vi "_ExecuteInstruction.vi"(2 "Telemetry":refnum<k21>, 4 "Instructions":refnum<k21>, 5 "Output":refnum<k21>, 6 "error in (no error)":errorcluster, 7 "DebugOut":refnum<k21>, 8 "Port":T1="Mod6\\Port1", 9 "MPU in":refnum<class "MPU.lvclass">) -> (0 "error out":errorcluster, 1 "End Loop":bool, 3 "MPU out":refnum<class "MPU.lvclass">)   [LabVIEW 2018, in "Modbus_Processing_Unit.lvlib" / "MPU.lvclass"]
uses:
  MPU.lvclass
  PortType.ctl
  MPU.lvclass/MPU.ctl
  <vilib>/rvi/DataTransferAndStorage/Container/Common/niFpgaContainerExecOnDevCompGetState.vi
  <vilib>/rvi/Emulation/niFpgaEmulationIsFPGAContextNoSignature.vi
  <vilib>/rvi/DataTransferAndStorage/Container/Common/niFpgaContainerGetUniqueNameForEmu.vi
  <vilib>/rvi/Emulation/niFpgaProcessEmulError.vi
  <vilib>/rvi/Emulation/niFpgaSctlEmulationGetInTimedLoop.vi
  <vilib>/rvi/errors/nirviReportUnexpectedCaseInternalError (U32).vi
  <vilib>/rvi/Memory/Memory_Emulation/niFpgaMemoryEmulationCacheClearOnFirstRun.vi
  <vilib>/rvi/Memory/Memory_Emulation/nirvimemoryEmulationManagerCache_MakeExclusive.vi
  <vilib>/rvi/Memory/Memory_Emulation/niFpgaMemoryEmulationValidateCache.vi
  <vilib>/rvi/Memory/Memory_Emulation/nirvimemoryEmulationManagerCache_InsertValue.vi
  <vilib>/Utility/error.llb/Clear Errors.vi
  <vilib>/rvi/Memory/Memory_Emulation/nirvimemoryEmulationManagerCache_ReleaseExclusive.vi
  <vilib>/rvi/Memory/Memory_Emulation/nirvimemoryEmulationManagerCache_GetValue.vi
  <vilib>/rvi/Memory/Memory_Emulation/nirvimemoryEmulationManagerCache_SetValue.vi
  <vilib>/rvi/Emulation/niFpgaSctlEmulationResourceMgr.vi
  <vilib>/rvi/errors/niFpgaSetErrorForExecOnDevCompSimple.vi
  <vilib>/rvi/eio/common/nirviEmuReportErrorAndStop.vi
  <vilib>/rvi/FIFO/Fifo_Resource/nirvififoEmulationSetSize.vi
  <vilib>/rvi/FIFO/Fifo_Resource/nirviFifoEmulationQueueMgr.vi
  <instcachedir>/0/nirviFifoEmulationQueueMgr_E5CAEC123FF24DC58D834DCA3CDAA9B5.lvgen/nirviFifoEmulationQueueMgr_E5CAEC123FF24DC58D834DCA3CDAA9B5_001.vi
  <vilib>/rvi/FIFO/Fifo_Resource/nirvififoEmulationDetermineInputValidOut.vi
  <vilib>/rvi/FIFO/Fifo_Resource/nirvififoEmulationCreateLock.vi
  <vilib>/rvi/FIFO/Fifo_Resource/nirvififoEmulationObtainLock.vi
  <vilib>/rvi/FIFO/Fifo_Resource/nirvififoEmulationReleaseLock.vi
  <vilib>/rvi/occurrence/nirviWaitOnOccurrenceBase.vi
  <vilib>/rvi/errors/nirviReportUnexpectedCaseInternalError.vi
  <vilib>/rvi/interface/RandomDataEmulation/niFpgaRandomDataHandleErrors.vi
  <vilib>/rvi/DataTransferAndStorage/Container/XNode/niFpgaContainer.xnode
  <vilib>/rvi/Memory/Memory_Emulation/niFpgaMemoryEmulationRefIn.vi
  <vilib>/rvi/FIFO/Fifo_Resource/niFpgaFifoEmulationRefIn.vi
panel:
  # "Excutes a single instruction. Modify IP as needed. Signal if \ninstruction reading loop shall end in End Loop indicator."
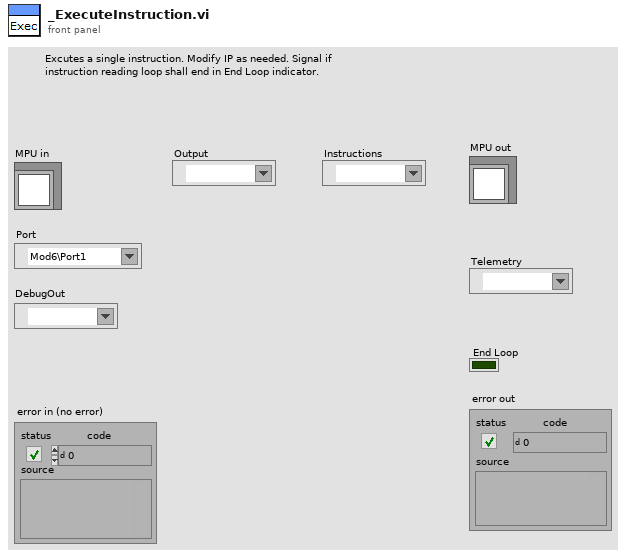
[diagram p1: front panel]
types:
  T1 = typedef "PortType.ctl" = refnum<k21>
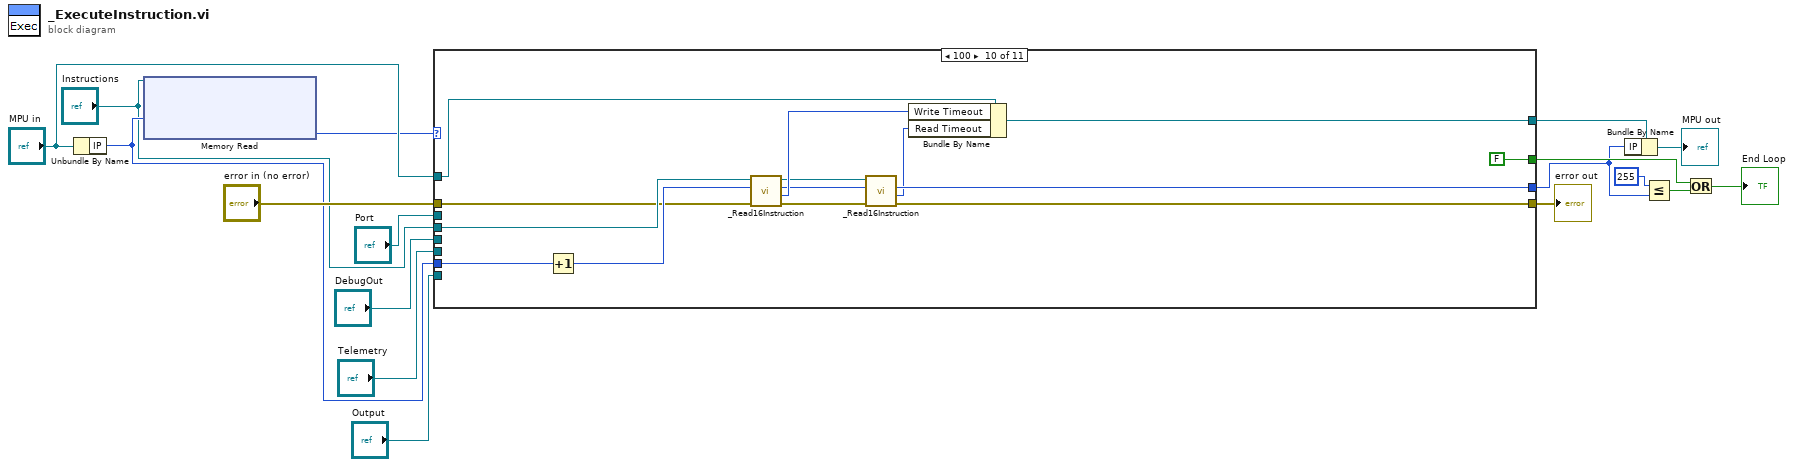
[diagram p0: block diagram]
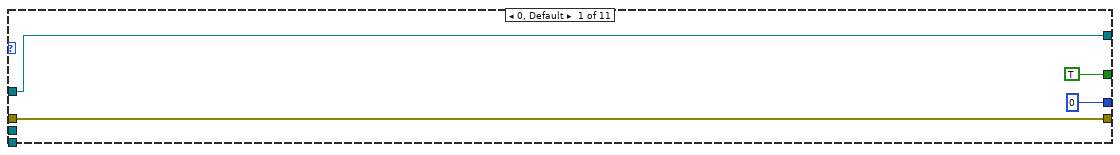
[diagram p2: hidden frame]
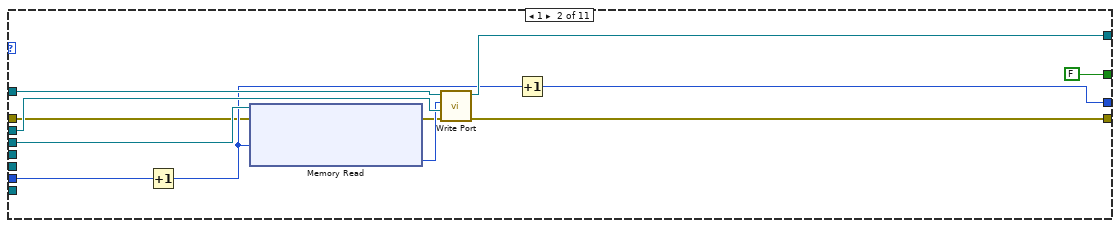
[diagram p3: hidden frame]
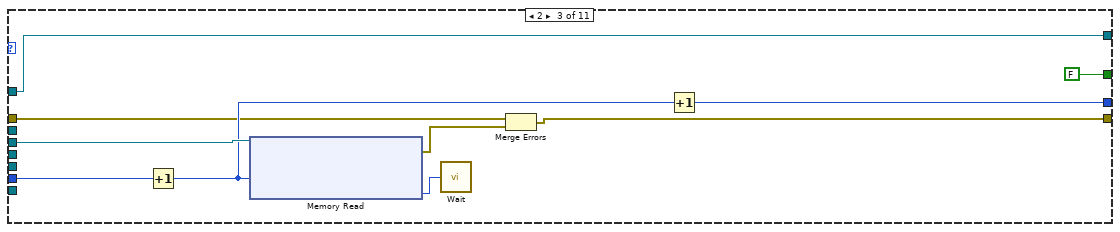
[diagram p4: hidden frame]
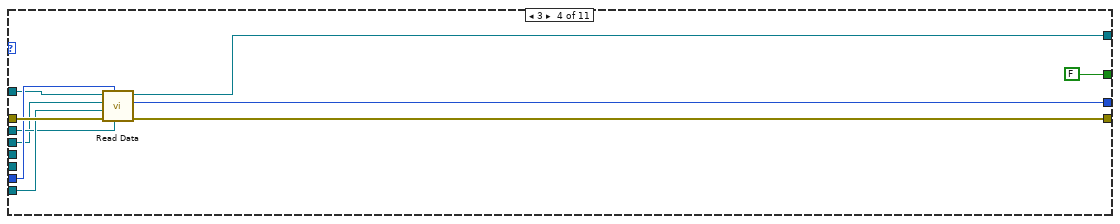
[diagram p5: hidden frame]
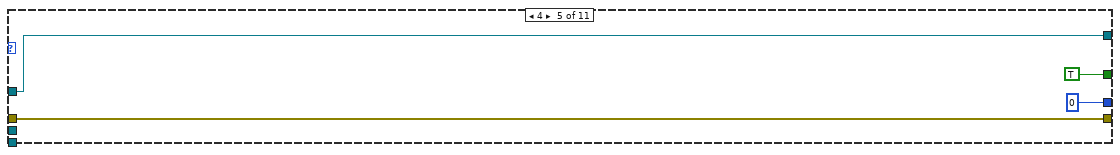
[diagram p6: hidden frame]
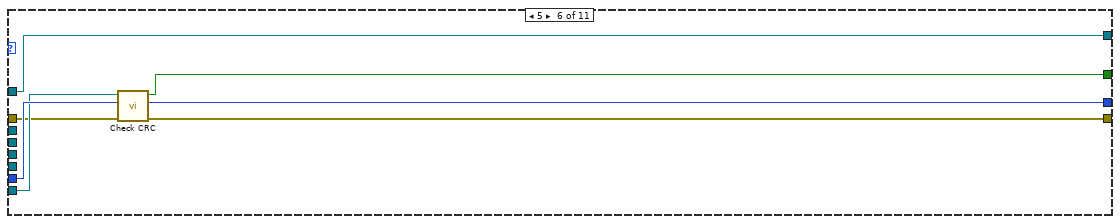
[diagram p7: hidden frame]
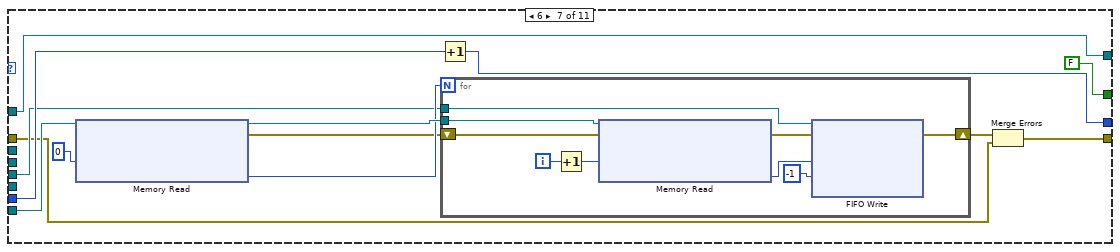
[diagram p8: hidden frame]
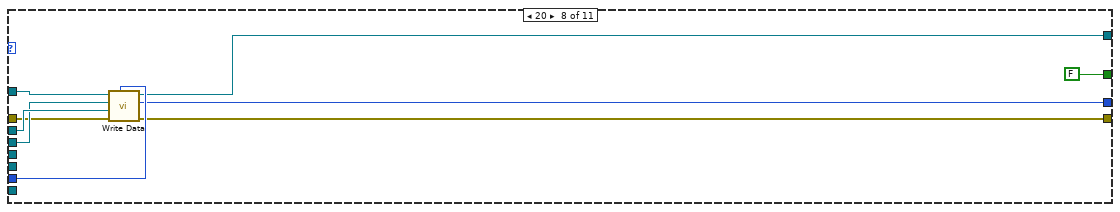
[diagram p9: hidden frame]
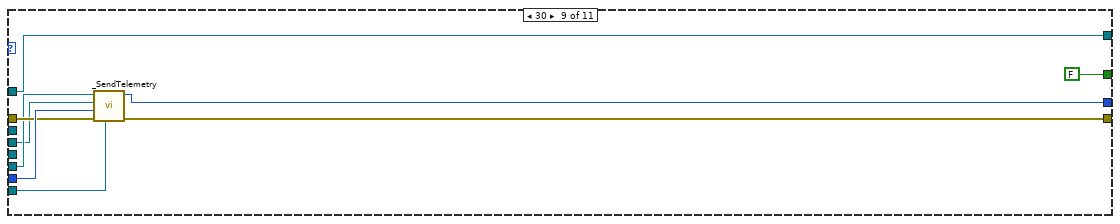
[diagram p10: hidden frame]
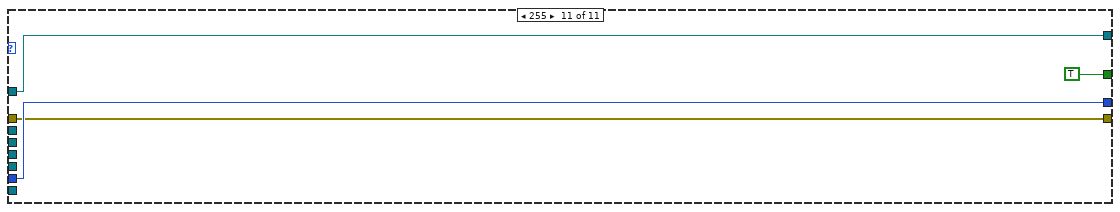
[diagram p11: hidden frame]
diagram:
  n1 = Unbundle By Name("MPU in") -> ("IP"=w5:i16)
  n2 = xnode ("Memory Read")("Address"=w5, "Memory In"="Instructions") -> ("Data"=w4:u8)  [unwired: 1 out]
  n3 = case shown="100" w4 {
    tunnel: [TRUE FALSE FALSE FALSE TRUE w60 FALSE FALSE FALSE FALSE ("Button") TRUE] -> w11
    tunnel: "error in (no error)" -> [w20 w23 w34 w52 w55 w58 w67 w89 w100 w112 w119]
    tunnel: w5 -> [_ w32 w43 w51 _ w63 w76 w94 w101 w116 w121]
    tunnel: [i16 0 ("IP") w31 w42 w53 i16 0 w62 w75 w92 w99 w108 w121] -> w10
    tunnel: "Output" -> [_ _ _ w49 _ w59 w73 _ w96 _ _]
    tunnel: [w20 w28 w35 w48 w55 w61 w68 w88 w103 w105 w119] -> w16
    tunnel: "MPU in" -> [w19 w30 w40 w46 w54 w64 w74 w95 w104 w118 w122]
    tunnel: [w19 w29 w40 w47 w54 w64 w74 w87 w104 w115 w122] -> w14
    tunnel: "Telemetry" -> [_ _ _ _ _ _ _ _ w98 _ _]
    tunnel: "Port" -> [_ w27 _ w45 _ _ _ w91 _ _ _]
    tunnel: "Instructions" -> [_ w26 w39 w44 _ _ _ w90 w97 w114 _]
    tunnel: "DebugOut" -> [_ _ _ _ _ _ w69 _ _ _ _]
    frame 0, Default {
    }
    frame 1 {
      n4 = Increment(x=w32) -> (x+1=w25:i16)
      n5 = xnode ("Memory Read")("Address"=w25, "error in (no error)"=w23, "Memory In"=w26) -> ("Data"=w24:u8, "error out"=w22:errorcluster)  [unwired: 1 out]
      n6 = call-dynamic "Write Port.vi"("error in (no error)"=w22, "Port"=w27, "Data"=w24, "MPU in"=w30) -> ("error out"=w28:errorcluster, "MPU out"=w29:refnum<class "MPU.lvclass">)  [unwired: 5 in, 1 out]
      n7 = Increment(x=w25) -> (x+1=w31:i16)
    }
    frame 2 {
      n8 = Increment(x=w43) -> (x+1=w36:i16)
      n9 = xnode ("Memory Read")("Address"=w36, "Memory In"=w39) -> ("Data"=w37:u8, "error out"=w38:errorcluster)  [unwired: 1 in, 1 out]
      n10 = call "Wait"("Count(mSec)"=w37) -> ()  [unwired: 1 out]
      n11 = Merge Errors(w34, w38) -> (w35:errorcluster)
      n12 = Increment(x=w36) -> (x+1=w42:i16)
    }
    frame 3 {
      n13 = call-dynamic "Read Data.vi"("Port"=w45, "IP"=w51, "error in (no error)"=w52, "Output"=w49, "Instructions"=w44, "MPU in"=w46) -> ("error out"=w48:errorcluster, "IP Out"=w53:i16, "MPU out"=w47:refnum<class "MPU.lvclass">)  [unwired: 3 in]
    }
    frame 4 {
    }
    frame 5 {
      n14 = call "Check CRC.vi"("error in (no error)"=w58, "IP"=w63, "Refnum in"=w59) -> ("error out"=w61:errorcluster, "Numeric"=w62:i16, "Button"=w60:bool)  [unwired: 6 in]
    }
    frame 6 {
      n15 = xnode ("Memory Read")("Address"=u32 0, "Memory In"=w73) -> ("Data"=w70:u8, "error out"=w66:errorcluster, "Memory Out"=w71:refnum<k21>)  [unwired: 1 in]
      n16 = Increment(x=w76) -> (x+1=w75:i16)
      n17 = for {
        N: w70 -> [_]
        tunnel: w69 -> [w86]
        tunnel: w71 -> [w84]
        shift-right: [w78] -> w65
        shift-left: w66 -> [w80]
        i -> [w83]
        n18 = Increment(x=w83) -> (x+1=w82:i32)
        n19 = xnode ("Memory Read")("Address"=w82, "error in (no error)"=w80, "Memory In"=w84) -> ("Data"=w81:u8, "error out"=w79:errorcluster)  [unwired: 1 out]
        n20 = xnode ("FIFO Write")("Element"=w81, "Timeout"=-1, "error in (no error)"=w79, "FIFO In"=w86) -> ("error out"=w78:errorcluster)  [unwired: 2 out]
      }
      n21 = Merge Errors(w65, w67) -> (w68:errorcluster)
    }
    frame 20 {
      n22 = call-dynamic "Write Data.vi"("IP"=w94, "error in (no error)"=w89, "Port"=w91, "Instructions"=w90, "MPU in"=w95) -> ("error out"=w88:errorcluster, "Numeric"=w92:i16, "MPU out"=w87:refnum<class "MPU.lvclass">)  [unwired: 4 in]
    }
    frame 30 {
      n23 = call "_SendTelemetry.vi"("Output"=w96, "error in (no error)"=w100, "IP in"=w101, "Instructions"=w97, "Telemetry FIFO"=w98) -> ("error out"=w103:errorcluster, "IP out"=w99:i16)  [unwired: 5 in]
    }
    frame 100 {
      n24 = Increment(x=w116) -> (x+1=w113:i16)
      n25 = call "_Read16Instruction.vi"("error in (no error)"=w112, "Address In"=w113, "Refnum in"=w114) -> ("error out"=w106:errorcluster, "Value"=w111:i16, "Address Out"=w110:i16, "Refnum Out"=w109:refnum<k21>)  [unwired: 3 in]
      n26 = call "_Read16Instruction.vi"("error in (no error)"=w106, "Address In"=w110, "Refnum in"=w109) -> ("error out"=w105:errorcluster, "Value"=w107:i16, "Address Out"=w108:i16)  [unwired: 3 in, 1 out]
      n27 = Bundle By Name(cluster=w118, "Write Timeout"=w111, "Read Timeout"=w107) -> (w115:refnum<class "MPU.lvclass">)
    }
    frame 255 {
    }
  }
  "error out" <- w16
  n28 = Bundle By Name(cluster=w14, "IP"=w10) -> (→"MPU out":refnum<class "MPU.lvclass">)
  n29 = Less Or Equal?(x=i16 255 ("y"), y=w10) -> (x <= y?=w9:bool)
  n30 = Or(x=w11, y=w9) -> (x .or. y?=→"End Loop":bool)
